vi "Write ACIR Setting.vi"(8 "error in (no error)":errorcluster, 10 "ACIR Setting":T1 {"Frequency" format="%#_6p"}, 11 "ACIR configuration":refnum<class "ACIR configuration.lvclass">) -> (0 "error out":errorcluster, 3 "ACIR configuration out":refnum<class "ACIR configuration.lvclass">)   [LabVIEW 2025, in "ACIR.lvlib" / "ACIR configuration.lvclass"]
uses:
  ACIR configuration.lvclass
  ACIR Instrument Setting.ctl
  ACIR configuration.lvclass/ACIR configuration.ctl
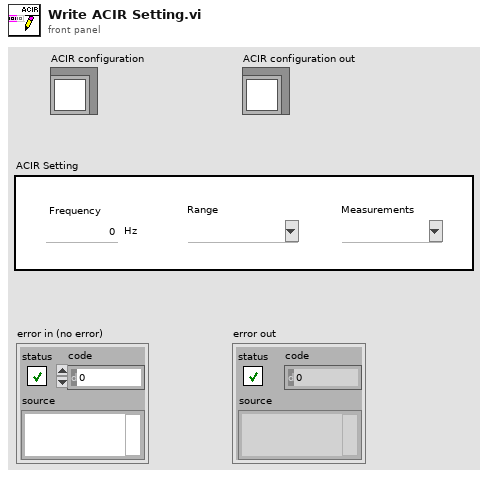
[diagram p1: front panel]
types:
  T1 = typedef "ACIR.lvlib/ACIR configuration.lvclass/ACIR Instrument Setting.ctl" = cluster{"Frequency":dbl, "Range":string, "Measurements":string}
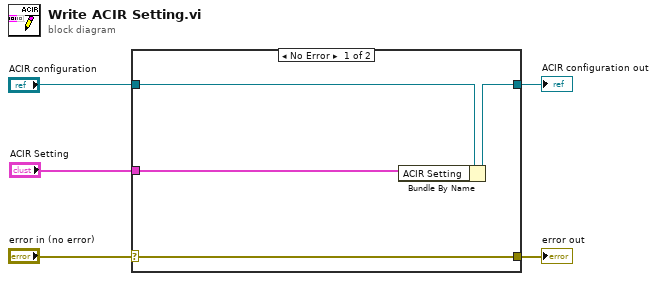
[diagram p0: block diagram]
diagram:
  n1 = case shown="No Error" "error in (no error)" {
    selector: "error in (no error)" -> [w9 w10]
    tunnel: [w9 w10] -> w4
    tunnel: [w7 w11] -> w2
    tunnel: "ACIR configuration" -> [w8 w11]
    tunnel: "ACIR Setting" -> [w6 _]
    frame No Error {
      n2 = Bundle By Name(cluster=w8, "ACIR Setting"=w6) -> (w7:refnum<class "ACIR configuration.lvclass">)
    }
    frame Error {
    }
  }
  "error out" <- w4
  "ACIR configuration out" <- w2
